vi "Parse JWT Elements.vi"(8 "error in (no error)":errorcluster, 11 "JSONWebToken in":refnum<class "JSONWebToken.lvclass">) -> (0 "error out":errorcluster, 3 "JSONWebToken out":refnum<class "JSONWebToken.lvclass">)   [LabVIEW 2024, in "JSONWebToken.lvclass"]
uses:
  JSONWebToken.lvclass
  JSONWebToken.lvclass/JSONWebToken.ctl
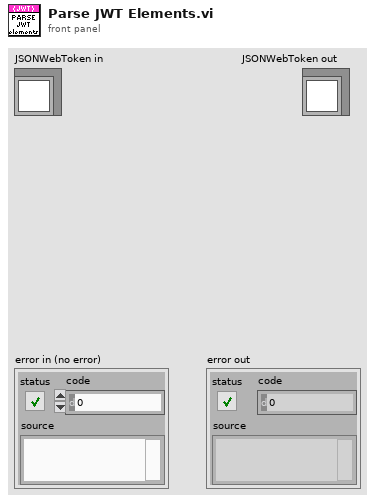
[diagram p1: front panel]
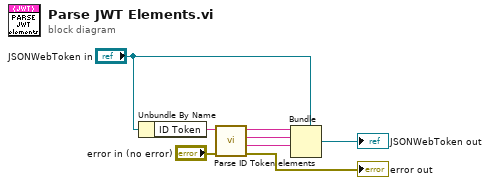
[diagram p0: block diagram]
diagram:
  n1 = Unbundle By Name("JSONWebToken in") -> ("ID Token"=w3:string)
  n2 = call "Parse ID Token elements.vi"("error in (no error)"="error in (no error)", "ID Token"=w3) -> ("error out"=→"error out":errorcluster, "signature"=w1:string, "payload"=w6:string, "header"=w5:string)  [unwired: 6 in]
  n3 = Bundle(cluster="JSONWebToken in", w5, w6, w1) -> (→"JSONWebToken out":refnum<class "JSONWebToken.lvclass">)  [unwired: 1 in]
